vi "HLine0005.vi"   [LabVIEW 2013]
uses:
  ModeType.ctl
  <vilib>/Heliosphere Research LLC/Advanced Plotting Toolkit/api_core/NewPlotScales.ctl
  <vilib>/Heliosphere Research LLC/Advanced Plotting Toolkit/Advanced Plotting Toolkit.lvlib
types:
  T1 = typedef "Advanced Plotting Toolkit.lvlib/NewPlotScales.ctl" = enum16{"Default", "Linear", "Log", "Symlog"}
  T2 = typedef "ModeType.ctl" = enum16{"Normal", "Expected Failure", "Skipped"}
  T3 = typedef "Advanced Plotting Toolkit.lvlib/PlotID.ctl" = i32
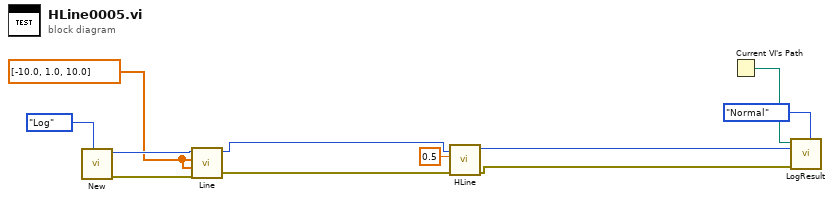
[diagram p0: block diagram]
diagram:
  w5 = dbl[] [-10.0, 1.0, 10.0] ("X Data")
  n1 = call <vilib>:"New.vi"("X Axis Scale"=NewPlotScales."Log") -> ("error out"=w6:errorcluster, "Plot ID"=w7:T3)  [unwired: 9 in]
  n2 = call <vilib>:"Line.vi"("error in (no error)"=w6, "Y Data"=w5, "X Data"=w5, "Plot ID"=w7) -> ("error out"=w1:errorcluster, "Plot ID out"=w2:T3)  [unwired: 6 in]
  n3 = call <vilib>:"HLine.vi"("error in (no error)"=w1, "Y (data coords)"=0.5, "Plot ID"=w2) -> ("error out"=w8:errorcluster, "Plot ID Out"=w9:T3)  [unwired: 7 in]
  n4 = Current VI's Path() -> (path=w11:path)
  n5 = call "LogResult.vi"("Mode"=ModeType."Normal", "Test Result"=w8, "Test Artifact"=w9, "VI Path"=w11) -> ()  [unwired: 8 in]
